vi "Post WebMessage.vi"(0 "Display State In":T1, 5 "Message":string, 7 "Send as JSON":bool, 9 "Container State":T2, 11 "error in (no error)":errorcluster) -> (4 "Display State Out":T1, 15 "error out":errorcluster)   [LabVIEW 2020, in "WebView2 Control.xctl"]
uses:
  WebView2 Control.xctl
  Webview2 Lib/WebView2 Control Object/WebView2 Control.lvclass
  <vilib>/_xctls/Container State.ctl
  <vilib>/_xctls/XControlSupport.lvlib
  State.ctl
panel:
  # "Add Controls & Indicators that form the parameters of the method here. Hook them to the connector pane. Do not delete the controls & indicators that are already hooked to the connector pane.\n \nTo setup the parameters  for this method, right click on this item in the Project Tree & select \"Configure Method...\"."
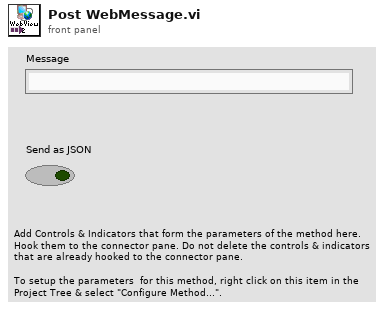
[diagram p1: front panel]
types:
  T1 = typedef "WebView2 Control.xctl/State.ctl" = cluster{"Control Object Ref":refnum<data-value>}
  T2 = typedef "XControlSupport.lvlib/Container State.ctl" = cluster{"Indicator?":bool, "Run Mode?":bool, " Refnum":refnum<vi>}
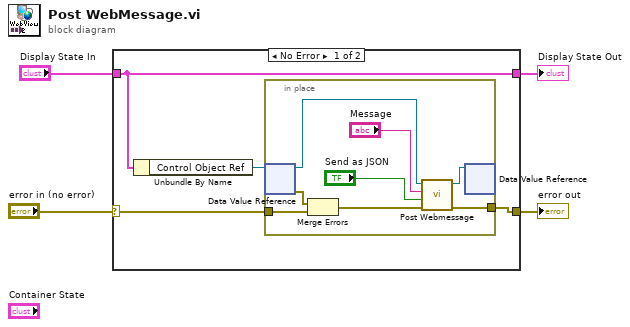
[diagram p0: block diagram]
diagram:
  n1 = case shown="No Error" "error in (no error)" {
    selector: "error in (no error)" -> [w5 w18]
    tunnel: [w6 w18] -> w3
    tunnel: "Display State In" -> [w8 w17]
    tunnel: [w8 w17] -> w1
    frame No Error {
      n2 = Unbundle By Name(w8) -> ("Control Object Ref"=w7:refnum<data-value>)
      n3 = in-place {
        in-place-border: [w12] -> w6
        in-place-border: w5 -> [w10]
        n4 = in-place-dvr #1(w7) -> (w16:refnum<class "WebView2 Control.lvclass">, w14:errorcluster)
        n5 = Merge Errors(w14, w10) -> (w11:errorcluster)
        n6 = call "Post Webmessage.vi"("error in (no error)"=w11, "Send as JSON"="Send as JSON", "Message"="Message", "WebView2 Control in"=w16) -> ("error out"=w12:errorcluster, "WebView2 Control out"=w13:refnum<class "WebView2 Control.lvclass">)  [unwired: 6 in]
        n7 = in-place-dvr #1(w13) -> ()  [unwired: 2 out]
      }
    }
    frame Error {
    }
  }
  "error out" <- w3
  "Display State Out" <- w1
